vi "DATA-IN-2LOGIC.vi"(2 "SIZE":i32, 3 "data IN":string) -> (0 "ANALOGICAS":string, 1 "LOGICAS":T1)   [LabVIEW 2010]
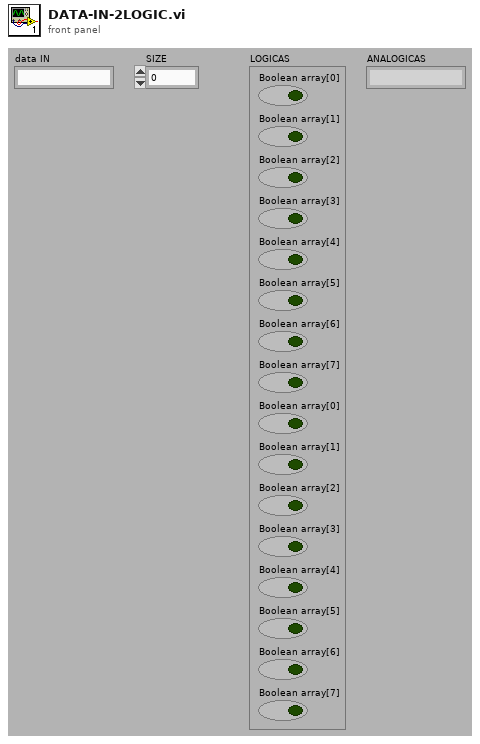
[diagram p1: front panel]
types:
  T1 = cluster{"Boolean array[0]":bool, "Boolean array[1]":bool, "Boolean array[2]":bool, "Boolean array[3]":bool, "Boolean array[4]":bool, "Boolean array[5]":bool, "Boolean array[6]":bool, "Boolean array[7]":bool, "Boolean array[0]":bool, "Boolean array[1]":bool, "Boolean array[2]":bool, "Boolean array[3]":bool, "Boolean array[4]":bool, "Boolean array[5]":bool, "Boolean array[6]":bool, "Boolean array[7]":bool}
  T2 = cluster{"unsigned byte array[0]":u8, "unsigned byte array[1]":u8}
  T3 = cluster{"Boolean array[0]":bool, "Boolean array[1]":bool, "Boolean array[2]":bool, "Boolean array[3]":bool, "Boolean array[4]":bool, "Boolean array[5]":bool, "Boolean array[6]":bool, "Boolean array[7]":bool}
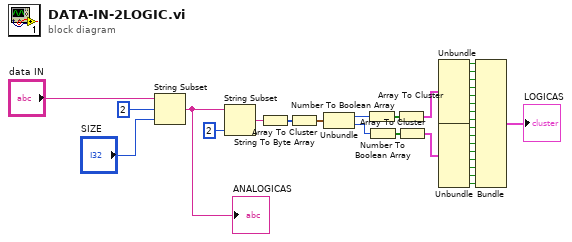
[diagram p0: block diagram]
diagram:
  n1 = String Subset(string="data IN", offset (0)=2, length (rest)="SIZE") -> (substring=w28:string)
  "ANALOGICAS" <- w28
  n2 = String Subset(string=w28, length (rest)=2 ("length (rest)")) -> (substring=w9:string)  [unwired: 1 in]
  n3 = String To Byte Array(string=w9) -> (unsigned byte array=w5:u8[])
  n4 = Array To Cluster(array=w5) -> (cluster=w6:T2)
  n5 = Unbundle(w6) -> ("unsigned byte array[0]"=w7:u8, "unsigned byte array[1]"=w30:u8)
  n6 = Number To Boolean Array(number=w7) -> (Boolean array=w8:bool[])
  n7 = Number To Boolean Array(number=w30) -> (Boolean array=w29:bool[])
  n8 = Array To Cluster(array=w8) -> (cluster=w15:T3)
  n9 = Array To Cluster(array=w29) -> (cluster=w31:T3)
  n10 = Unbundle(w15) -> ("Boolean array[0]"=w18:bool, "Boolean array[1]"=w14:bool, "Boolean array[2]"=w13:bool, "Boolean array[3]"=w12:bool, "Boolean array[4]"=w11:bool, "Boolean array[5]"=w10:bool, "Boolean array[6]"=w16:bool, "Boolean array[7]"=w17:bool)
  n11 = Unbundle(w31) -> ("Boolean array[0]"=w19:bool, "Boolean array[1]"=w20:bool, "Boolean array[2]"=w21:bool, "Boolean array[3]"=w22:bool, "Boolean array[4]"=w23:bool, "Boolean array[5]"=w24:bool, "Boolean array[6]"=w25:bool, "Boolean array[7]"=w26:bool)
  n12 = Bundle("Boolean array[0]"=w18, "Boolean array[1]"=w14, "Boolean array[2]"=w13, "Boolean array[3]"=w12, "Boolean array[4]"=w11, "Boolean array[5]"=w10, "Boolean array[6]"=w16, "Boolean array[7]"=w17, "Boolean array[0]"=w19, "Boolean array[1]"=w20, "Boolean array[2]"=w21, "Boolean array[3]"=w22, "Boolean array[4]"=w23, "Boolean array[5]"=w24, "Boolean array[6]"=w25, "Boolean array[7]"=w26) -> (→"LOGICAS":T1)  [unwired: 1 out]
